vi "BoolCmd_Send_Internal.vi"(7 "Command Name":string, 11 "Value":bool=TRUE) -> (0 "error out":errorcluster)   [LabVIEW 2019, in "Trajectory_Library.lvlib"]
uses:
  Trajectory_Library.lvlib
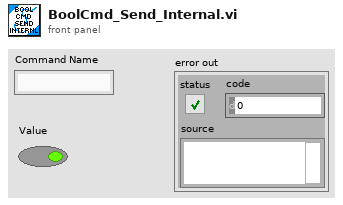
[diagram p1: front panel]
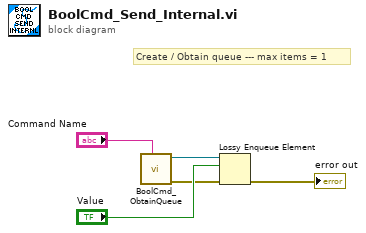
[diagram p0: block diagram]
diagram:
  # "Create / Obtain queue --- max items = 1"
  n1 = call "BoolCmd_ObtainQueue.vi"("Command Name"="Command Name") -> ("error out"=w3:errorcluster, "Queue out"=w5:refnum<queue>)  [unwired: 9 in]
  n2 = Lossy Enqueue Element(queue=w5, element="Value", error in (no error)=w3) -> (error out=→"error out":errorcluster)  [unwired: 3 out]
